vi "CommPortPopup.vi"() -> (0 "error out":errorcluster, 3 "VISA resource name out":refnum<visa-resource-name>)   [LabVIEW 2015]
uses:
  <vilib>/Instr/_visa.llb/VISA Configure Serial Port (Instr).vi
panel:
  in  "Cancel":bool
  in  "OK Button":bool
  in  "Serial Communications Port":refnum<visa-resource-name>
  # "Select Comm Port"
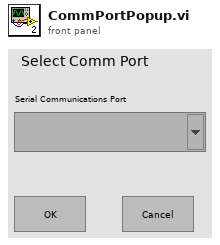
[diagram p1: front panel]
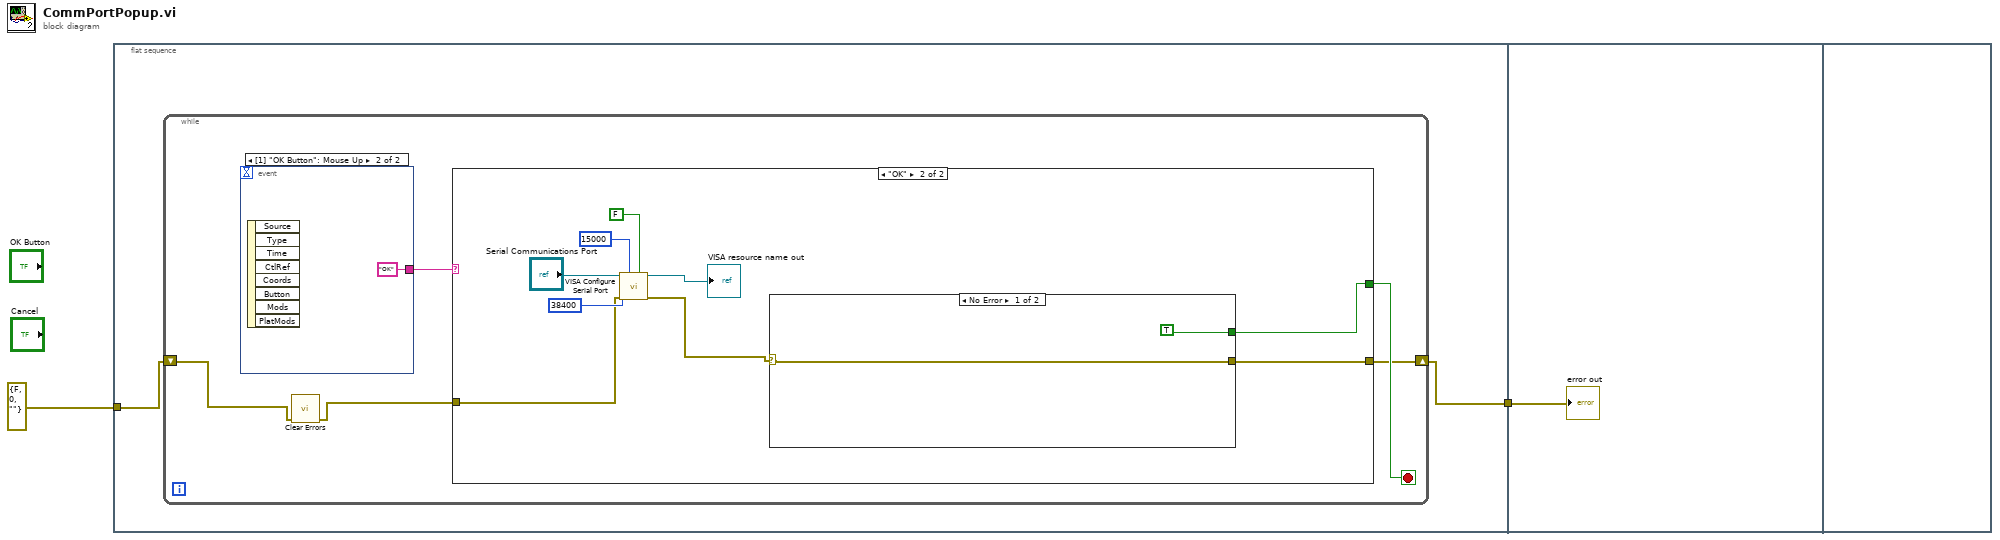
[diagram p0: block diagram]
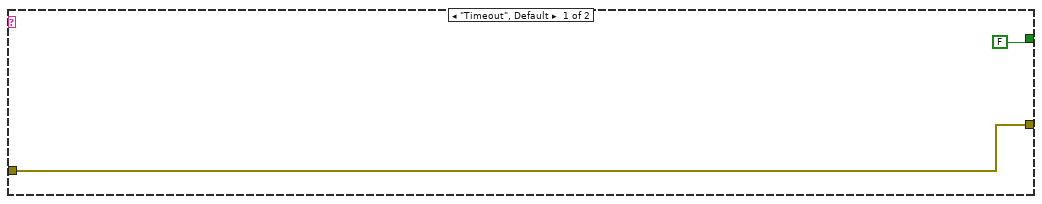
[diagram p2: hidden frame]
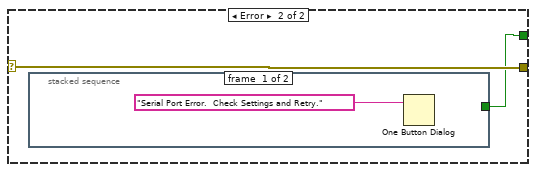
[diagram p3: hidden frame]
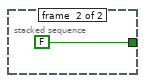
[diagram p4: hidden frame]
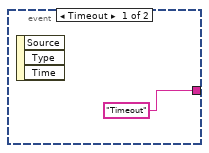
[diagram p5: hidden frame]
diagram:
  n1 = flat-sequence {
    tunnel: errorcluster {"status"=FALSE, "code"=0, "source"=""} ("error in (no error)") -> [w4]
    tunnel: [w3] -> w1
    tunnel: w1 -> [w29]
    frame #0 {
      n2 = while {
        shift-right: [w7] -> w3
        shift-left: w4 -> [w6]
        stop <- w8 stop-if-true
        n3 = event shown="[1] \"OK Button\": Mouse Up" {
          selector: _ -> [_ _]
          dyn-events: _ -> [_ _]
          timeout: _ -> [_ _]
          tunnel: ["Timeout" "OK"] -> w9
          event Timeout {
            n4 = event-data() -> ()  [unwired: 1 in, 3 out]
          }
          event "OK Button": Mouse Up {
            n5 = event-data() -> ()  [unwired: 1 in, 8 out]
          }
        }
        n6 = call <vilib>:"Clear Errors.vi"("error in (no error)"=w6) -> ("error out"=w5:errorcluster)  [unwired: 5 in, 1 out]
        n7 = case shown="\"OK\"" w9 {
          tunnel: [FALSE w14] -> w8
          tunnel: [w10 w13] -> w7
          tunnel: w5 -> [w10 w12]
          frame "Timeout", Default {
          }
          frame "OK" {
            n8 = call-poly "VISA Configure Serial Port"("VISA resource name"="Serial Communications Port", "timeout (10sec)"=u32 15000, "Enable Termination\nChar (T)"=FALSE ("Enable Termination\nChar (T)"), "baud rate (9600)"=u32 38400, "error in (no error)"=w12) -> ("VISA resource name out"=→"VISA resource name out":refnum<visa-resource-name>, "error out"=w15:errorcluster)  [unwired: 9 in]
            n9 = case shown="No Error" w15 {
              selector: w15 -> [w21 w24]
              tunnel: [w21 w24] -> w13
              tunnel: [TRUE w23] -> w14
              frame No Error {
              }
              frame Error {
                n10 = stacked-sequence {
                  tunnel: [_ FALSE] -> w23
                  frame #0 {
                    n11 = One Button Dialog(message="Serial Port Error.  Check Settings and Retry.") -> ()  [unwired: 1 in, 1 out]
                  }
                  frame #1 {
                  }
                }
              }
            }
          }
        }
      }
    }
    frame #1 {
      "error out" <- w29
    }
    frame #2 {
    }
  }
